vi "Combined Server no CRDS or PAS.vi"   [LabVIEW 2012]
uses:
  Reusable/Serial IO/Serial IO.lvclass
  Devices/CLAP/CLAP.lvclass
  <vilib>/DAQmx/write.llb/DAQmx Write (Digital 1D Bool NChan 1Samp 1Line).vi
  <vilib>/DAQmx/miscellaneous.llb/DAQmx Fill In Error Info.vi
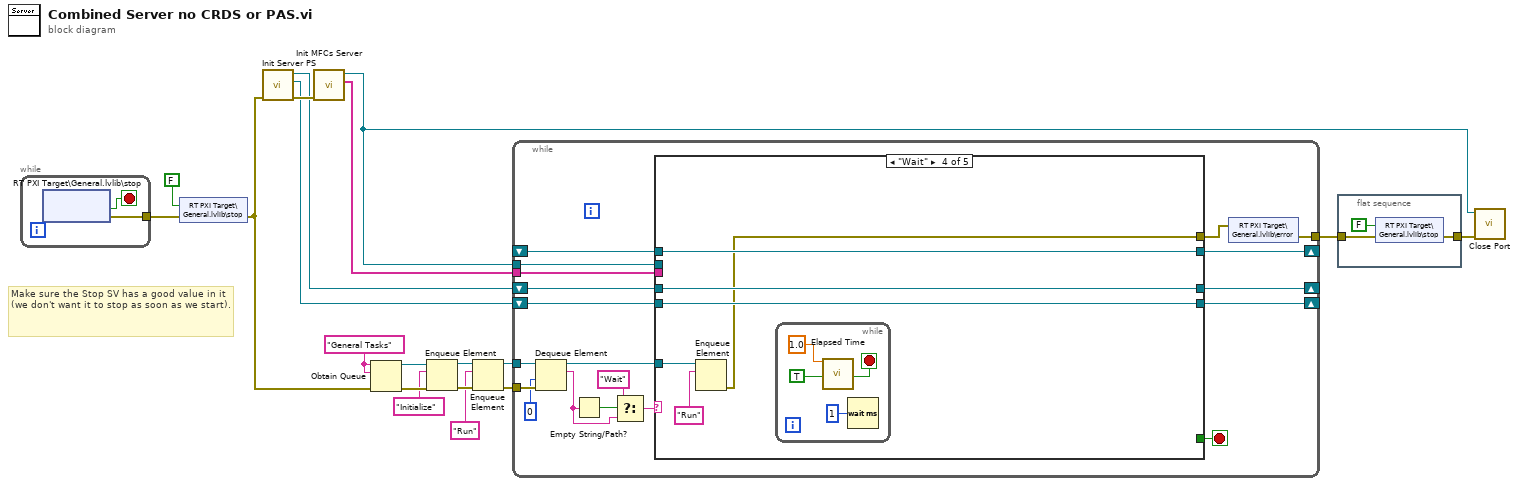
[diagram p0: block diagram]
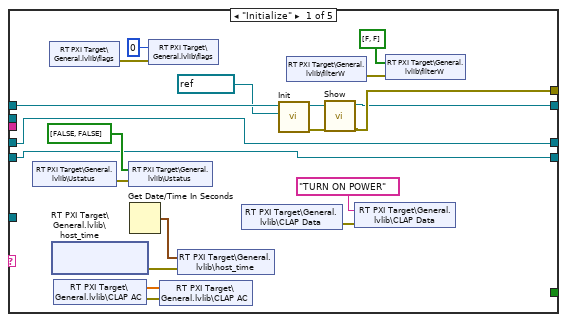
[diagram p2: hidden frame]
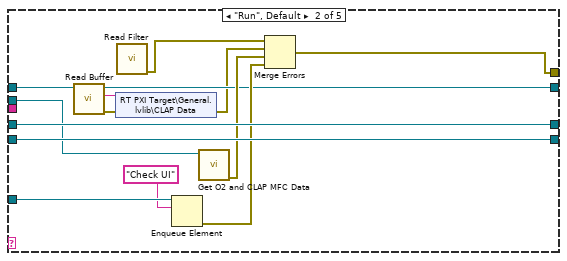
[diagram p3: hidden frame]
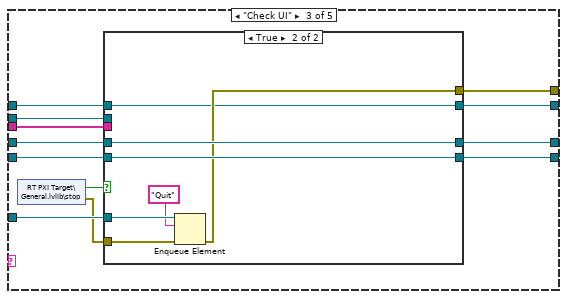
[diagram p4: hidden frame]
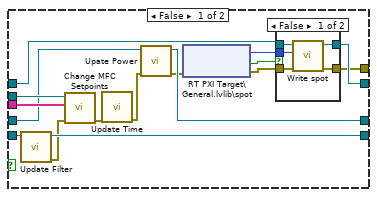
[diagram p5: hidden frame]
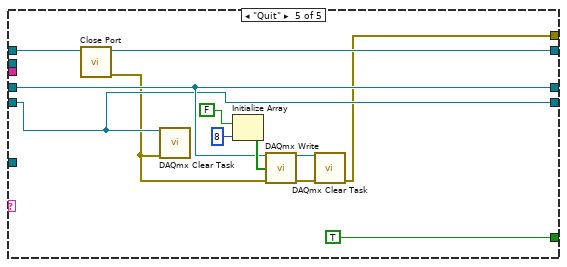
[diagram p7: hidden frame]
diagram:
  w10 = "General Tasks" ("name (unnamed)")
  # "Make sure the Stop SV has a good value in it (we don't want it to stop as soon as we start)."
  n1 = while {
    tunnel: [w20] -> w18
    stop <- w21 stop-if-true
    n2 = shared-variable "RT PXI Target\\General.lvlib\\stop"() -> (error out=w20:errorcluster, w21:bool)  [unwired: 2 in, 1 out]
  }
  n3 = shared-variable "RT PXI Target\\General.lvlib\\stop"(FALSE ("stop"), error in=w18) -> (error out=w15:errorcluster)
  n4 = call "Init Server PS.vi"("error in"=w15) -> ("error out"=w14:errorcluster, "Filter Out Task"=w13:refnum<k21>, "PS Switch Out"=w12:refnum<k21>)  [unwired: 8 in]
  n5 = call "Init MFCs Server.vi"("error in"=w14) -> ("Address Out"=w16:string[], "Serial IO out"=w1:refnum<class "Serial IO.lvclass">)  [unwired: 8 in, 1 out]
  n6 = Obtain Queue(name (unnamed)=w10, element data type=w10, error in (no error)=w15) -> (queue out=w9:refnum<queue>, error out=w8:errorcluster)  [unwired: 2 in, 1 out]
  n7 = Enqueue Element(queue=w9, element="Initialize", error in (no error)=w8) -> (queue out=w6:refnum<queue>, error out=w5:errorcluster)  [unwired: 1 in, 1 out]
  n8 = Enqueue Element(queue=w6, element="Run", error in (no error)=w5) -> (queue out=w3:refnum<queue>, error out=w4:errorcluster)  [unwired: 1 in, 1 out]
  n9 = while {
    tunnel: w1 -> [w38]
    tunnel: w16 -> [w37]
    tunnel: w4 -> [w33]
    tunnel: w3 -> [w34]
    shift-right: [w35] -> _
    shift-left: w13 -> [w36]
    shift-right: [w39] -> _
    shift-left: w12 -> [w40]
    shift-right: [w27] -> _
    shift-left: _ -> [w26]
    tunnel: [w22] -> w11
    stop <- w25 stop-if-true
    n10 = Dequeue Element(queue=w34, timeout in ms (-1)=0, error in (no error)=w33) -> (queue out=w28:refnum<queue>, element=w31:string)  [unwired: 2 out]
    n11 = Empty String/Path?(string/path=w31) -> (empty?=w32:bool)
    n12 = Select(t="Wait", s=w32, f=w31) -> (s? t:f=w29:string)
    n13 = case shown="\"Wait\"" w29 {
      tunnel: [w42 w68 w77 w117 w128] -> w23
      tunnel: w40 -> [w51 w72 w82 w121 w131]
      tunnel: [w51 w72 w80 w121 w131] -> w39
      tunnel: w38 -> [_ w70 w83 _ _]
      tunnel: w37 -> [_ _ w84 _ _]
      tunnel: w36 -> [w50 w71 w86 w120 w130]
      tunnel: [w50 w71 w85 w120 w130] -> w35
      tunnel: w28 -> [_ w74 w81 w119 _]
      tunnel: [w41 w64 w78 w122 w137] -> w27
      tunnel: w26 -> [w60 w65 w79 w122 w138]
      tunnel: [_ _ _ _ TRUE] -> w25
      frame "Initialize" {
        n14 = shared-variable "RT PXI Target\\General.lvlib\\Ustatus"() -> (error out=w57:errorcluster)  [unwired: 1 in, 1 out]
        n15 = shared-variable "RT PXI Target\\General.lvlib\\flags"() -> (error out=w54:errorcluster)  [unwired: 1 in, 1 out]
        n16 = shared-variable "RT PXI Target\\General.lvlib\\host_time"() -> (error out=w55:errorcluster)  [unwired: 2 in, 2 out]
        n17 = shared-variable "RT PXI Target\\General.lvlib\\CLAP AC"() -> (w46:sgl[], error out=w47:errorcluster)  [unwired: 1 in]
        n18 = shared-variable "RT PXI Target\\General.lvlib\\Ustatus"(bool[] [FALSE, FALSE], error in=w57) -> ()  [unwired: 1 out]
        n19 = Get Date/Time In Seconds() -> (seconds since 1Jan1904=w56:timestamp)
        n20 = shared-variable "RT PXI Target\\General.lvlib\\flags"(u8 0 ("flags"), error in=w54) -> ()  [unwired: 1 out]
        n21 = shared-variable "RT PXI Target\\General.lvlib\\CLAP AC"(w46, error in=w47) -> ()  [unwired: 1 out]
        n22 = shared-variable "RT PXI Target\\General.lvlib\\host_time"(w56, error in=w55) -> ()  [unwired: 1 out]
        n23 = shared-variable "RT PXI Target\\General.lvlib\\CLAP Data"() -> (error out=w49:errorcluster)  [unwired: 1 in, 1 out]
        n24 = call-dynamic "Init.vi"("Port"=refnum<visa-resource-name> "CLAP", "CLAP in"=w60) -> ("error out"=w43:errorcluster, "CLAP out"=w44:refnum<class "CLAP.lvclass">)  [unwired: 8 in]
        n25 = shared-variable "RT PXI Target\\General.lvlib\\filterW"() -> (error out=w53:errorcluster)  [unwired: 1 in, 1 out]
        n26 = call "Show.vi"("error in"=w43, "CLAP in"=w44) -> ("error out"=w42:errorcluster, "CLAP out"=w41:refnum<class "CLAP.lvclass">)  [unwired: 8 in]
        n27 = shared-variable "RT PXI Target\\General.lvlib\\CLAP Data"("TURN ON POWER" ("CLAP Data"), error in=w49) -> ()  [unwired: 1 out]
        n28 = shared-variable "RT PXI Target\\General.lvlib\\filterW"(bool[] [FALSE, FALSE] ("filterW"), error in=w53) -> ()  [unwired: 1 out]
      }
      frame "Run", Default {
        n29 = call "Read Buffer.vi"("CLAP in"=w65) -> ("error out"=w62:errorcluster, "Buffer"=w63:string, "CLAP out"=w64:refnum<class "CLAP.lvclass">)  [unwired: 8 in]
        n30 = shared-variable "RT PXI Target\\General.lvlib\\CLAP Data"(w63, error in=w62) -> (error out=w61:errorcluster)
        n31 = call "Read Filter.vi"() -> ("error out"=w69:errorcluster)  [unwired: 11 in]
        n32 = Enqueue Element(queue=w74, element="Check UI") -> (error out=w67:errorcluster)  [unwired: 2 in, 2 out]
        n33 = call "Get O2 and CLAP MFC Data.vi"("Serial IO in"=w70) -> ("error out"=w66:errorcluster)  [unwired: 10 in]
        n34 = Merge Errors(w69, w61, w66, w67) -> (w68:errorcluster)
      }
      frame "Check UI" {
        n35 = shared-variable "RT PXI Target\\General.lvlib\\stop"() -> (w75:bool, error out=w76:errorcluster)  [unwired: 1 in]
        n36 = case shown="True" w75 {
          tunnel: w86 -> [w102 w113]
          tunnel: [w101 w113] -> w85
          tunnel: w84 -> [w100 _]
          tunnel: w83 -> [w99 _]
          tunnel: w82 -> [w98 w114]
          tunnel: w81 -> [_ w116]
          tunnel: [w97 w114] -> w80
          tunnel: w79 -> [w96 w110]
          tunnel: [w95 w110] -> w78
          tunnel: [w94 w111] -> w77
          tunnel: w76 -> [_ w112]
          frame False {
            n37 = call "Update Filter.vi"("Refnum in"=w102) -> ("error out"=w93:errorcluster, "Refnum out"=w101:refnum<k21>)  [unwired: 9 in]
            n38 = call "Change MFC Setpoints.vi"("error in"=w93, "Address Out"=w100, "Serial IO in"=w99) -> ("error out"=w92:errorcluster)  [unwired: 7 in, 1 out]
            n39 = call "Update Time.vi"("error in"=w92) -> ("error out"=w91:errorcluster)  [unwired: 10 in]
            n40 = call "Upate Power.vi"("error in"=w91, "Refnum in"=w98) -> ("error out"=w90:errorcluster, "Refnum out"=w97:refnum<k21>)  [unwired: 8 in]
            n41 = shared-variable "RT PXI Target\\General.lvlib\\spot"(error in=w90) -> (w88:u8, error out=w89:errorcluster, w87:bool)  [unwired: 1 in]
            n42 = case shown="False" w87 {
              tunnel: w96 -> [w107 w108]
              tunnel: [w106 w108] -> w95
              tunnel: [w105 w109] -> w94
              tunnel: w89 -> [w104 w109]
              tunnel: w88 -> [w103 _]
              frame False {
                n43 = call-dynamic "Write spot.vi"("error in"=w104, "spot"=w103, "CLAP in"=w107) -> ("error out"=w105:errorcluster, "CLAP out"=w106:refnum<class "CLAP.lvclass">)  [unwired: 7 in]
              }
              frame True {
              }
            }
          }
          frame True {
            n44 = Enqueue Element(queue=w116, element="Quit", error in (no error)=w112) -> (error out=w111:errorcluster)  [unwired: 1 in, 2 out]
          }
        }
      }
      frame "Wait" {
        n45 = Enqueue Element(queue=w119, element="Run") -> (error out=w117:errorcluster)  [unwired: 2 in, 2 out]
        n46 = while {
          stop <- w126 stop-if-true
          n47 = call "Elapsed Time"("Time Target (s)"=1.0, "Auto Reset"=TRUE) -> ("Time has Elapsed"=w126:bool)  [unwired: 10 in, 7 out]
          n48 = Wait (ms)(milliseconds to wait=u32 1) -> ()  [unwired: 1 out]
        }
      }
      frame "Quit" {
        n49 = call-dynamic "Close Port.vi"("CLAP in"=w138) -> ("error out"=w129:errorcluster, "CLAP out"=w137:refnum<class "CLAP.lvclass">)  [unwired: 9 in]
        n50 = call <vilib>:"DAQmx Clear Task.vi"("task in"=w130, "error in"=w129) -> ()  [unwired: 13 in, 1 out]
        n51 = Initialize Array(FALSE, 8 ("dimension size")) -> (w134:bool[])
        n52 = call-poly <vilib>:"DAQmx Write.vi"("task/channels in"=w131, "data"=w134, "error in"=w129) -> ("task out"=w135:refnum<k21>, "error out"=w136:errorcluster)  [unwired: 10 in, 1 out]
        n53 = call <vilib>:"DAQmx Clear Task.vi"("task in"=w135, "error in"=w136) -> ("error out"=w128:errorcluster)  [unwired: 13 in]
      }
    }
    n54 = shared-variable "RT PXI Target\\General.lvlib\\error"(w23) -> (error out=w22:errorcluster)  [unwired: 1 in]
  }
  n55 = flat-sequence {
    tunnel: w11 -> [w140]
    tunnel: [w139] -> w17
    frame #0 {
      n56 = shared-variable "RT PXI Target\\General.lvlib\\stop"(FALSE ("stop"), error in=w140) -> (error out=w139:errorcluster)
    }
  }
  n57 = call-dynamic "Close Port.vi"("error in (no error)"=w17, "Serial IO in"=w1) -> ()  [unwired: 8 in, 2 out]
